vi "Overlay Ellipse Axes.vi"(10 "array":dbl[](array[numeric]), 11 "Image Out":T1) -> (3 "Image Out 2":T1)   [LabVIEW 2011]
uses:
  <vilib>/vision/Image Controls.llb/IMAQ Image.ctl
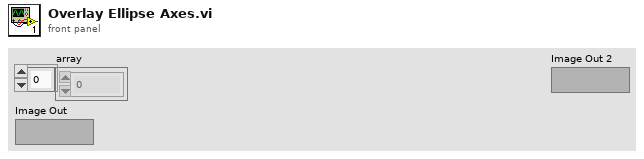
[diagram p1: front panel]
types:
  T1 = typedef "IMAQ Image.ctl" = refnum<image>
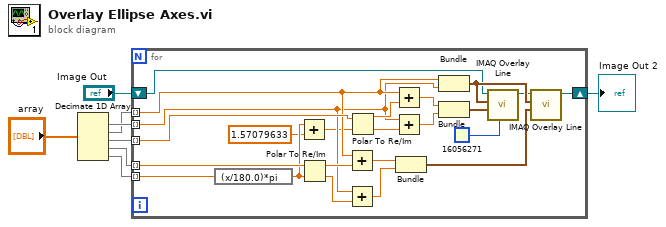
[diagram p0: block diagram]
diagram:
  n1 = Decimate 1D Array("array") -> (w6:dbl[], w5:dbl[], w8:dbl[], w4:dbl[], w7:dbl[])  [unwired: 1 out]
  n2 = for {
    tunnel: w8 -> [w31] mode=indexing
    tunnel: w7 -> [w15] mode=indexing
    tunnel: w6 -> [w20] mode=indexing
    tunnel: w5 -> [w21] mode=indexing
    shift-right: [w10] -> w1
    shift-left: "Image Out" -> [w9]
    tunnel: w4 -> [w24] mode=indexing
    n3 = expression code="(x/180.0)*pi" ("degrees to radians")(w15) -> (w14:dbl)
    n4 = Add(x=w14, y=1.57079633) -> (x+y=w13:dbl)
    n5 = Polar To Re/Im(2:w14, 3:w24) -> (0:w22:dbl, 1:w23:dbl)
    n6 = Add(x=w21, y=w23) -> (x+y=w18:dbl)
    n7 = Add(x=w20, y=w22) -> (x+y=w19:dbl)
    n8 = Polar To Re/Im(2:w13, 3:w31) -> (0:w29:dbl, 1:w30:dbl)
    n9 = Add(x=w21, y=w30) -> (x+y=w28:dbl)
    n10 = Add(x=w20, y=w29) -> (x+y=w27:dbl)
    n11 = Bundle(w18, w19) -> (w17:cluster{dbl, dbl})  [unwired: 1 in]
    n12 = Bundle(w21, w20) -> (w16:cluster{dbl, dbl})  [unwired: 1 in]
    n13 = Bundle(w28, w27) -> (w26:cluster{dbl, dbl})  [unwired: 1 in]
    n14 = call "IMAQ Overlay Line"("Color"=u32 16056271, "End Point"=w26, "Start Point"=w16, "Image"=w9) -> ("Image Out"=w11:T1)  [unwired: 6 in, 1 out]
    n15 = call "IMAQ Overlay Line"("End Point"=w17, "Start Point"=w16, "Image"=w11) -> ("Image Out"=w10:T1)  [unwired: 7 in, 1 out]
  }
  "Image Out 2" <- w1
